vi "U32 Color To Hexa String.vi"(10 "U32 Color":u32(colorbox)) -> (2 "8 Char Hexa String":string)   [LabVIEW 2021, in "Appearance Actor.lvlib" / "Generic Theme.lvclass"]
doc: "Converts U32 to 8 char hexa string."
uses:
  Generic Theme.lvclass
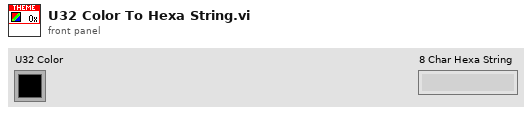
[diagram p1: front panel]
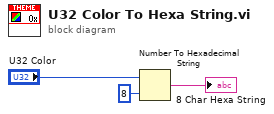
[diagram p0: block diagram]
diagram:
  n1 = Number To Hexadecimal String(1:i16 8 ("width (-)"), 2:"U32 Color") -> (0:→"8 Char Hexa String":string)
